vi "convertHexToDecimal.vi"(8 "error in (no error)":errorcluster, 10 "hexString":string, 11 "EncoderReader in":refnum<class "EncoderReader.lvclass">) -> (0 "error out":errorcluster, 1 "checksumOKIsTrue":bool, 2 "decimalValue":i32, 3 "EncoderReader out":refnum<class "EncoderReader.lvclass">)   [LabVIEW 2013, in "EncoderReader.lvclass"]
uses:
  EncoderReader.lvclass
panel:
  out "stringValue":string
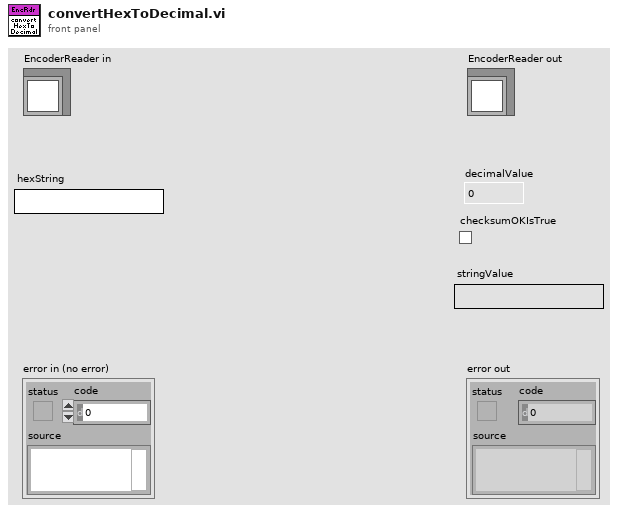
[diagram p1: front panel]
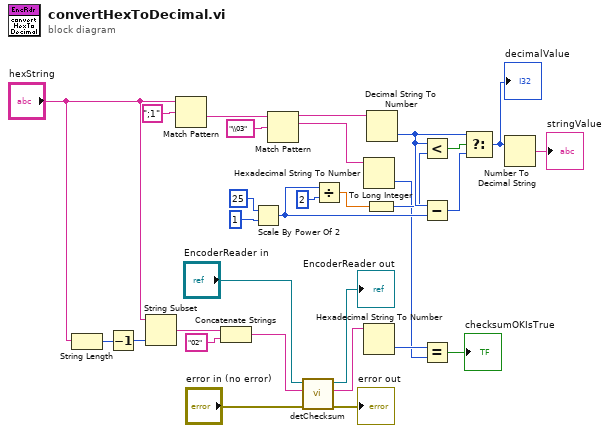
[diagram p0: block diagram]
diagram:
  n1 = String Length(string="hexString") -> (length=w15:i32)
  n2 = Decrement(x=w15) -> (x-1=w14:i32)
  n3 = String Subset(string="hexString", length (rest)=w14) -> (substring=w11:string)  [unwired: 1 out]
  n4 = Match Pattern(string="hexString", regular expression=";1") -> (after substring=w30:string)  [unwired: 4 out]
  n5 = Concatenate Strings(w11, "02") -> (w12:string)
  n6 = Scale By Power Of 2(n=25, x=1) -> (x*2^n=w20:i32)
  n7 = Match Pattern(string=w30, regular expression="\\03") -> (before substring=w29:string, match substring=w8:string)  [unwired: 3 out]
  n8 = call "detChecksum.vi"("error in (no error)"="error in (no error)", "inputString"=w12, "EncoderReader in"="EncoderReader in") -> ("error out"=→"error out":errorcluster, "checksumString"=w9:string, "EncoderReader out"=→"EncoderReader out":refnum<class "EncoderReader.lvclass">)  [unwired: 6 in]
  n9 = Divide(x=w20, y=2 ("x")) -> (x/y=w22:dbl)
  n10 = Hexadecimal String To Number(string=w8) -> (number=w6:u32)  [unwired: 3 out]
  n11 = Hexadecimal String To Number(string=w9) -> (number=w7:u32)  [unwired: 3 out]
  n12 = To Long Integer(number=w22) -> (32bit integer=w21:i32)
  n13 = Decimal String To Number(string=w29) -> (number=w27:i32)  [unwired: 3 out]
  n14 = Less?(x=w27, y=w21) -> (x < y?=w28:bool)
  n15 = Subtract(x=w27, y=w20) -> (x-y=w26:i32)
  n16 = Equal?(x=w7, y=w6) -> (x = y?=→"checksumOKIsTrue":bool)
  n17 = Select(t=w27, s=w28, f=w26) -> (s? t:f=w25:i32)
  "decimalValue" <- w25
  n18 = Number To Decimal String(number=w25) -> (decimal integer string=→"stringValue":string)  [unwired: 1 out]
